vi "20newsgroups.vi"(8 "error in (no error)":errorcluster caption="entrée d'erreur (pas d'erreur)", 11 "fetch_20newsgroups":T1={"subset"="train", "categories"=["None"], "shuffle"=TRUE, "random_state"=42, "remove"=[], "download_if_missing"=TRUE, "Returns"="Data"} {"random_state" min=-1}) -> (0 "error out":errorcluster, 3 "Data":string)   [LabVIEW 2020]
doc: "The 20 newsgroups dataset comprises around 18000 newsgroups posts on 20 topics split in two subsets: one for training (or development) and the other one for testing (or for performance evaluation). The split between the train and test set is based upon a messages posted before and after a specific date.\n\nThis module contains two loaders. The first one, sklearn.datasets.fetch_20newsgroups, returns a list of the raw texts that can be fed to text feature extractors such as sklearn.feature_extraction.text.CountVectorizer with custom parameters so as to extract feature vectors. The second one, sklearn.datasets.fetch_20newsgroups_vectorized, returns ready-to-use features, i.e., it is not necessary to use a feature extractor.\n\nData Set Characteristics :\n - Classes : 20\n - Samples total : 18846\n - Dimensionality : 1\n - Features : text\nParameters :\n\n- subset : ‘train’ or ‘test’, ‘all’, optional\nSelect the dataset to load: ‘train’ for the training set, ‘test’ for the test set, ‘all’ for both, with shuffled ordering.\n\n- categories : None or collection of string or unicode\nIf None (default), load all the categories. If not None, list of category names to load (other categories ignored).\n\n- shuffle : bool, optional\nWhether or not to shuffle the data: might be important for models that make the assumption that the samples are independent and identically distributed (i.i.d.), such as stochastic gradient descent.\n\n- random_state : int, RandomState instance, default=-1=None\nDetermines random number generation for dataset shuffling. Pass an int for reproducible output across multiple function calls. See Glossary.\n\n- remove : tuple\nMay contain any subset of (‘headers’, ‘footers’, ‘quotes’). Each of these are kinds of text that will be detected and removed from the newsgroup posts, preventing classifiers from overfitting on metadata.\n\n‘headers’ removes newsgroup headers, ‘footers’ removes blocks at the ends of posts that look like signatures, and ‘quotes’ removes lines that appear to be quoting another post.\n\n‘headers’ follows an exact standard; the other filters are not always correct.\n\n- download_if_missing : optional, True by default\nIf False, raise an IOError if the data is not locally available instead of trying to download the data from the source site.\n\n\nReturns : \n\n- data : list, length [n_samples]\n The data list to learn.\n\n- target : array, shape [n_samples]\nThe target labels."
uses:
  20newsgroups.lvclass
panel:
  out "20newsgroups.lvclass":refnum<class "20newsgroups.lvclass">
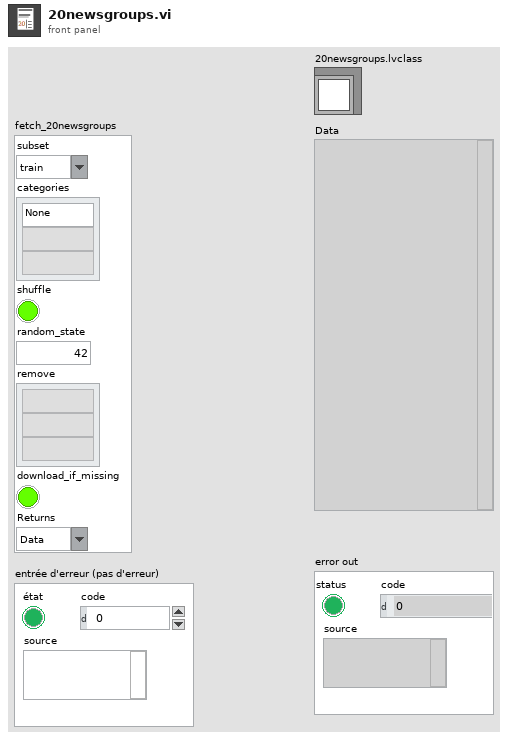
[diagram p1: front panel]
types:
  T1 = cluster{"subset":string, "categories":string[], "shuffle":bool, "random_state":i32, "remove":string[], "download_if_missing":bool, "Returns":string}
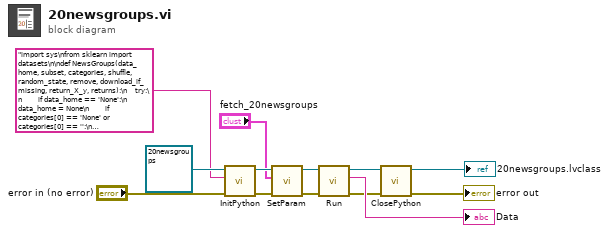
[diagram p0: block diagram]
diagram:
  n1 = call-dynamic "InitPython.vi"("error in (no error)"="error in (no error)", "Python Instruction"="import sys\nfrom sklearn import datasets\n\ndef NewsGroups(data_home, subset, categories, shuffle, random_state, remove, download_if_missing, return_X_y, returns):\n    try:\n        if data_home == 'None':\n            data_home = None\n        if categories[0] == 'None' or categories[0] == '':\n            categories = None\n        if random_state == -1:\n            random_state = None\n        remove = tuple(remove)\n        NewsGroups = datasets.fetch_20newsgroups(data_home, subset, categories, shuffle, random_state, remove, download_if_missing, return_X_y)\n        if returns == 'Data':\n            data = NewsGroups['data']\n            return str(data)\n        else :\n            data = NewsGroups['target'].tolist()\n            return str(data)  \n    except:\n        erreur = sys.exc_info()\n        typerr = u\"%s\" % (erreur[0])\n        typerr = typerr[typerr.find(\"'\")+1:typerr.rfind(\"'\")]\n        msgerr = u\"%s\" % (erreur[1])\n        message = str('//!\\\\ {0} : {1}'. format(typerr,msgerr))\n        return message", "Scikit-learn en entrée"=refnum<class "20newsgroups.lvclass"> refnum ("20newsgroups.lvclass")) -> ("error out"=w8:errorcluster, "Scikit-learn en sortie"=w9:refnum<class "20newsgroups.lvclass">)  [unwired: 7 in]
  n2 = call-dynamic "SetParam.vi"("error in (no error)"=w8, "fetch_20newsgroups"="fetch_20newsgroups", "20newsgroups.lvclass"=w9) -> ("error out"=w5:errorcluster, "20newsgroups.lvclass 2"=w6:refnum<class "20newsgroups.lvclass">)  [unwired: 7 in]
  n3 = call-dynamic "Run.vi"("error in (no error)"=w5, "20newsgroups.lvclass"=w6) -> ("error out"=w2:errorcluster, "Data"=→"Data":string, "20newsgroups.lvclass 2"=w4:refnum<class "20newsgroups.lvclass">)  [unwired: 7 in]
  n4 = call-dynamic "ClosePython.vi"("error in (no error)"=w2, "Scikit-learn en entrée"=w4) -> ("error out"=→"error out":errorcluster, "Scikit-learn en sortie"=→"20newsgroups.lvclass":refnum<class "20newsgroups.lvclass">)  [unwired: 8 in]
